vi "练习1.3-连续采集.vi"() -> ()   [LabVIEW 2021]
panel:
  in  "stop":bool
  out "Waveform Graph":dynamicdata(graph)
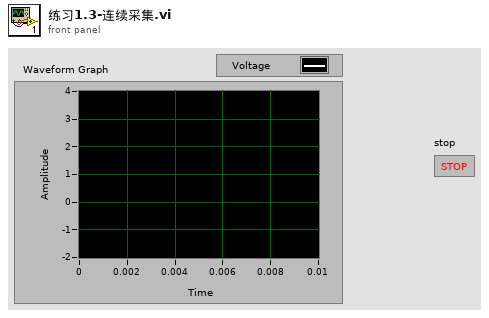
[diagram p1: front panel]
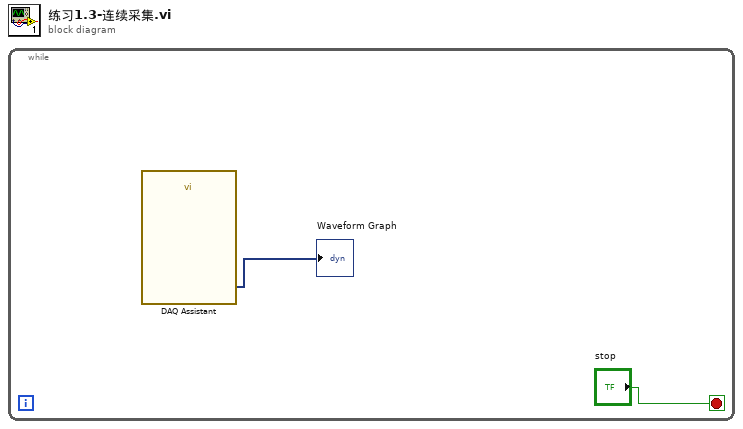
[diagram p0: block diagram]
diagram:
  n1 = while {
    stop <- "stop" stop-if-true
    n2 = call "DAQ Assistant"() -> ("data"=→"Waveform Graph":dynamicdata)  [unwired: 16 in, 3 out]
  }
